vi "FPGA Get P2P FIFO Endpoint By Name.vi"(8 "error in (no error)":errorcluster, 10 "FIFO":string, 11 "FPGA Session In":refnum<class "FPGA Interface Base.lvclass">) -> (0 "error out":errorcluster, 1 "Endpoint":u32, 3 "FPGA Session Out":refnum<class "FPGA Interface Base.lvclass">)   [LabVIEW 2010, in "FPGA Interface Base.lvclass"]
doc: "Gets an endpoint reference to a peer-to-peer FIFO."
uses:
  <userlib>/_FPGA Interface Advanced Tools/FPGA Interface Base/FPGA Interface Base.lvclass
  <userlib>/_FPGA Interface Advanced Tools/FPGA Interface Base/FPGA Interface Base.lvclass/FPGA Interface Base.ctl
  <vilib>/Utility/error.llb/Error Cluster From Error Code.vi
  <userlib>/_FPGA Interface Advanced Tools/FPGA Interface Base/Accessors/FPGA Read Session.vi
  <userlib>/_FPGA Interface Advanced Tools/FPGA Interface Wrapper/FPGA Interface Wrapper.lvlib
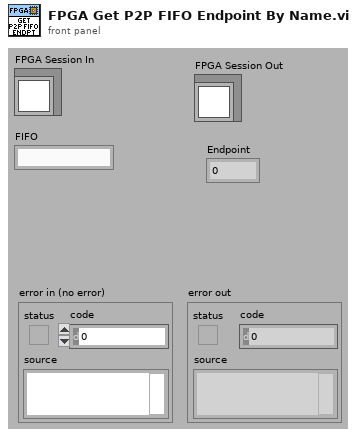
[diagram p1: front panel]
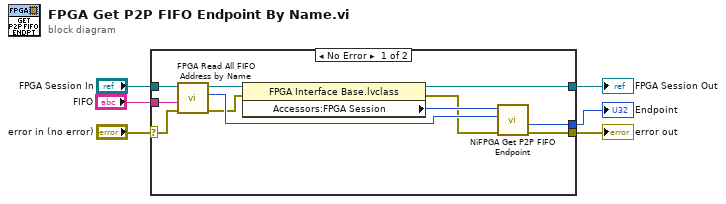
[diagram p0: block diagram]
diagram:
  n1 = case shown="No Error" "error in (no error)" {
    selector: "error in (no error)" -> [w16 w19]
    tunnel: [w8 w19] -> w2
    tunnel: [w9 w18] -> w3
    tunnel: "FPGA Session In" -> [w17 w18]
    tunnel: "FIFO" -> [w15 _]
    tunnel: [w7 _] -> w1
    frame No Error {
      n2 = call <userlib>:"FPGA Read All FIFO Address by Name.vi"("error in (no error)"=w16, "Name"=w15, "FPGA Interface Base in"=w17) -> ("error out"=w12:errorcluster, "Address"=w14:u32, "FPGA Interface Base out"=w13:refnum<class "FPGA Interface Base.lvclass">)  [unwired: 5 in, 1 out]
      n3 = property class="FPGA Interface Base.lvclass"(reference=w13, error in=w12) -> (reference out=w9:refnum<class "FPGA Interface Base.lvclass">, error out=w10:errorcluster, "Accessors:FPGA Session"=w11:u32)
      n4 = call <userlib>:"NiFPGA Get P2P FIFO Endpoint.vi"("error in (no error)"=w10, "FIFO"=w14, "Session"=w11) -> ("error out"=w8:errorcluster, "Endpoint"=w7:u32)  [unwired: 6 in, 1 out]
    }
    frame Error {
    }
  }
  "error out" <- w2
  "FPGA Session Out" <- w3
  "Endpoint" <- w1
